vi "DataGraph_Calc_Rectangle_X.vi"(9 "Minimum X":dbl, 10 "Maximum X":dbl, 11 "Raw X Array":dbl[](array[numeric])) -> (0 "Minimum Value":dbl format="%#_13g", 1 "Maximum Value":dbl format="%#_13g", 2 "Minimum Index":u32, 3 "Maximum Index":u32)   [LabVIEW 2018, in "DataGraphXControl.xctl"]
uses:
  DataGraphXControl.xctl
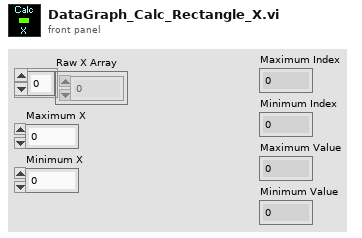
[diagram p1: front panel]
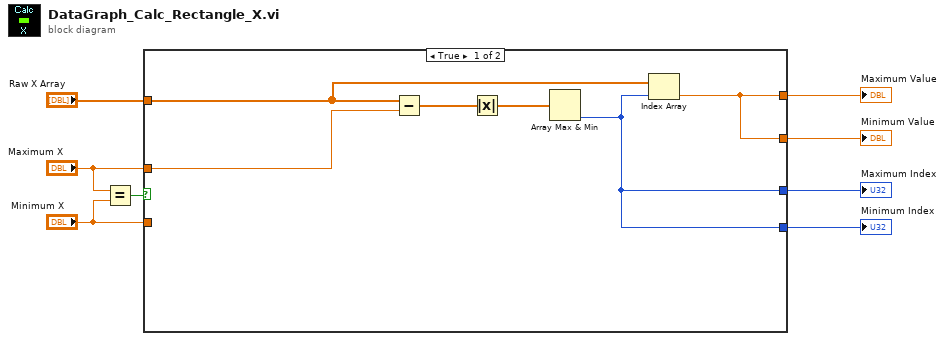
[diagram p0: block diagram]
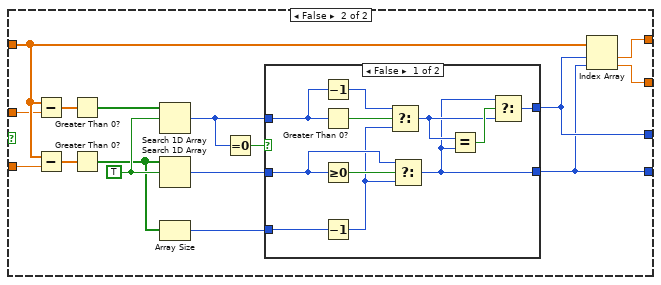
[diagram p2: hidden frame]
diagram:
  n1 = Equal?(x="Maximum X", y="Minimum X") -> (x = y?=w1:bool)
  n2 = case shown="True" w1 {
    tunnel: "Raw X Array" -> [w11 w23]
    tunnel: [w10 w22] -> w7
    tunnel: [w10 w21] -> w6
    tunnel: [w9 w20] -> w5
    tunnel: [w9 w19] -> w4
    tunnel: "Maximum X" -> [w13 w16]
    tunnel: "Minimum X" -> [_ w15]
    frame True {
      n3 = Subtract(x=w11, y=w13) -> (x-y=w14:dbl[])
      n4 = Absolute Value(x=w14) -> (abs(x)=w12:dbl[])
      n5 = Array Max & Min(array=w12) -> (min index (indices)=w9:i32)  [unwired: 3 out]
      n6 = Index Array(array=w11, index=w9) -> (element=w10:dbl)
    }
    frame False {
      w27 = TRUE
      n7 = Subtract(x=w23, y=w16) -> (x-y=w30:dbl[])
      n8 = Subtract(x=w23, y=w15) -> (x-y=w29:dbl[])
      n9 = Greater Than 0?(x=w30) -> (x > 0?=w28:bool[])
      n10 = Greater Than 0?(x=w29) -> (x > 0?=w26:bool[])
      n11 = Search 1D Array(1D array=w28, element=w27) -> (index of element=w18:i32)  [unwired: 1 in]
      n12 = Search 1D Array(1D array=w26, element=w27) -> (index of element=w24:i32)  [unwired: 1 in]
      n13 = Array Size(array=w26) -> (size(s)=w25:i32)
      n14 = Equal To 0?(x=w18) -> (x = 0?=w17:bool)
      n15 = case shown="False" w17 {
        tunnel: w25 -> [w40 _]
        tunnel: w24 -> [w37 _]
        tunnel: [w33 _] -> w20
        tunnel: [w32 _] -> w19
        tunnel: w18 -> [w31 _]
        frame False {
          n16 = Decrement(x=w31) -> (x-1=w39:i32)
          n17 = Greater Than 0?(x=w31) -> (x > 0?=w41:bool)
          n18 = Greater Or Equal To 0?(x=w37) -> (x >= 0?=w38:bool)
          n19 = Decrement(x=w40) -> (x-1=w36:i32)
          n20 = Select(t=w39, s=w41, f=w36) -> (s? t:f=w34:i32)
          n21 = Select(t=w37, s=w38, f=w36) -> (s? t:f=w32:i32)
          n22 = Equal?(x=w34, y=w32) -> (x = y?=w35:bool)
          n23 = Select(t=w32, s=w35, f=w34) -> (s? t:f=w33:i32)
        }
        frame True {
        }
      }
      n24 = Index Array(array=w23, index #1=w20, index #2=w19) -> (element #1=w22:dbl, element #2=w21:dbl)
    }
  }
  "Minimum Index" <- w4
  "Maximum Index" <- w5
  "Maximum Value" <- w7
  "Minimum Value" <- w6
